vi "Configure IR High Limit Query.vi"(7 "Mode":u16(ring) items=["IR"], 8 "error in (no error)":errorcluster, 10 "Step":T1=1 min=1 max=99 step=1, 11 "VISA resource name":refnum<visa-resource-name>) -> (0 "error out":errorcluster, 2 "IR Hi limit value [ohm]":string, 3 "VISA resource name out":refnum<visa-resource-name>)   [LabVIEW 2025, in "Chroma 19052.lvlib"]
uses:
  <instrlib>/Chroma 19052/Public/Utility/Type Def/steps--numeric.ctl
  <instrlib>/Chroma 19052/Chroma 19052.lvlib
panel:
  # "IR High Limit query"
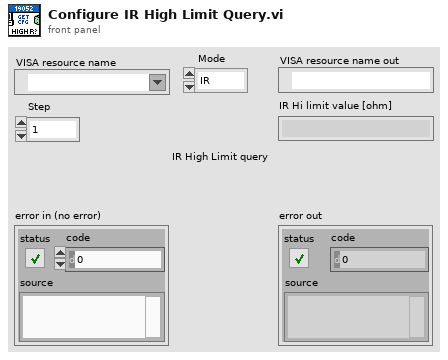
[diagram p1: front panel]
types:
  T1 = typedef "Chroma 19052.lvlib/steps--numeric.ctl" = u8
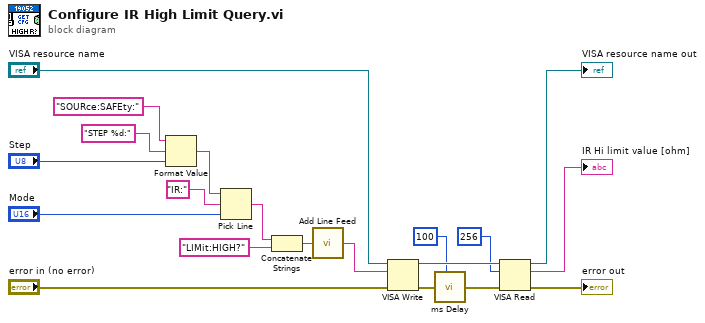
[diagram p0: block diagram]
diagram:
  n1 = Format Value(string ("")="SOURce:SAFEty:", format string="STEP %d:", value (0)="Step") -> (output string=w14:string)
  n2 = Pick Line(string ("")=w14, multi-line string="IR:", line index="Mode") -> (output string=w12:string)
  n3 = Concatenate Strings(w12, "LIMit:HIGH?" ("format string")) -> (w11:string)
  n4 = call <instrlib>:"Add Line Feed.vi"("Command string"=w11) -> ("Concatenated string"=w6:string)  [unwired: 4 in]
  n5 = VISA Write(VISA resource name="VISA resource name", write buffer=w6, error in (no error)="error in (no error)") -> (VISA resource name out=w20:refnum<visa-resource-name>, error out=w2:errorcluster)  [unwired: 1 out]
  n6 = call <instrlib>:"ms Delay.vi"("miliseconds to wait"=u32 100 ("Time Delay ms"), "error in (no error)"=w2) -> ("error out"=w3:errorcluster)  [unwired: 6 in, 1 out]
  n7 = VISA Read(VISA resource name=w20, byte count=u32 256, error in (no error)=w3) -> (VISA resource name out=→"VISA resource name out":refnum<visa-resource-name>, read buffer=→"IR Hi limit value [ohm]":string, error out=→"error out":errorcluster)  [unwired: 1 out]
